vi "PH_Timing.set Default.vi"(0 "i ref in":refnum<vi>, 5 "error in (no error)":errorcluster) -> (14 "i ref out":refnum<vi>, 19 "error out":errorcluster)   [LabVIEW 2014, in "PH_Timing.lvlib"]
doc: "Within this VI the default settings are set to the GUI."
uses:
  PH_Timing.lvlib
  PH_Basics/PH_Common/PH_Common.lvlib
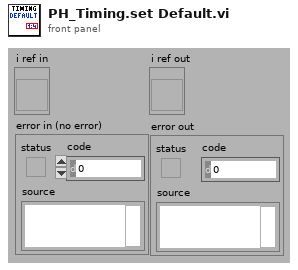
[diagram p1: front panel]
types:
  T1 = typedef "PH_Timing.lvlib/PH_Timing.i attribute.ctl" = cluster{"Sequencer":cluster{"linked?":bool, "Proc State":string, "Ref State":refnum<vi>}, "Gate Generator":cluster{"GD":cluster{"Device Status":T2, "linked?":bool}, "Settings":T3, "GUI Ref":refnum<vi>}, "Interlock Bypass":cluster{"Instancename":string, "Switch linked?":bool, "Device Status":T2, "Ref Status":refnum<vi>}, "Roughtuner":cluster{"Settings":T4, "GUI Ref":refnum<vi>, "GD":cluster{"Device Status":T2, "linked?":bool}}, "0,5Hz Gater":cluster{"Settings":T5, "GUI Ref":refnum<vi>, "GD":cluster{"Device Status":T2, "linked?":bool}}, "Slow Trigger":cluster{"Settings":T6, "GUI Ref":refnum<vi>, "Service ID Delay":i32, "Service ID Ext Trig":i32, "Wanted Settings":T6}, "Timing Mode":cluster{"Mode":T7, "GUI Ref":refnum<vi>, "Service ID T2":i32, "Service ID Mode":i32, "Wanted Mode":T7}, "ns Generator":cluster{"Settings":T8, "ns Generator Settings":refnum<vi>, "GD":cluster{"Device Status":T2, "linked?":bool}}, "Phase FEs":cluster{"Settings":T11, "GUI Ref":refnum<vi>, "Service ID Phase":i32, "Wanted Settings":T11}, "GD GUI Refs":refnum<vi>[], "Heads":T12[], "GUI Ref Delete":refnum<vi>}
  T2 = typedef "PH_StatusHandler.lvlib/PH_StatusHandler.Status.ctl" = i16
  T3 = typedef "PH_Timing.lvlib/PH_Timing.GateGen.ctl" = cluster{"Instance":string, "Channel Gate":i32, "Channel T2":i32, "Width Gate":dbl, "Width T2":dbl, "Delay Gate":dbl, "Delay T2":dbl, "Gate activ":bool, "T2 activ":bool, "System Mode":enum16{"Normal", "Single", "Burst", "Duty Cycle"}}
  T4 = typedef "PH_Timing.lvlib/PH_Timing.Roughtuner.ctl" = cluster{"Instance":string, "Phase PHELIX / UNILAC":cluster{"Channel":u16, "relative to":u16, "Delay [ms]":dbl}, "Pulse Length":cluster{"Channel":u16, "relative to":u16, "Delay [ms]":dbl}, "Trigger":cluster{"externally?":bool, "Rate [Hz]":dbl}}
  T5 = typedef "PH_Timing.lvlib/PH_Timing.0.5HzGater.ctl" = cluster{"Instance":string, "Channel ns FE Delay":i32, "Channel 0.5Hz":i32, "Width ns FE Delay":dbl, "Width 0.5Hz":dbl, "Delay ns FE Delay":dbl, "Delay 0.5Hz":dbl, "ns FE Delay active":bool, "0.5Hz activ":bool, "ns FE Delay inverted":bool, "0.5Hz inverted":bool}
  T6 = typedef "PH_Timing.lvlib/PH_Timing.Slow Trigger Settings.ctl" = cluster{"Delay":dbl, "externally triggered?":bool}
  T7 = typedef "PH_Timing.lvlib/PH_Timing.Timing Mode.ctl" = cluster{"T2":i16, "Modeselector":enum32{"10 Hz", "0.5 Hz", "Shot"}}
  T8 = typedef "PH_Timing.lvlib/PH_Timing.ns Generator.ctl" = cluster{"Instance":string, "Phase fs / ns FE":cluster{"Channel":T9, "Settings":T10}}
  T9 = typedef "Stanford Research DG645 - Driver.lvlib/Channel.ctl" = i32
  T10 = typedef "PH_SRDG645.lvlib/PH_SRDG645.Channel Settings.ctl" = cluster{"Delay [s]":dbl, "relative to":i32}
  T11 = typedef "PH_Timing.lvlib/PH_Timing.Phase FEs.ctl" = cluster{"Phase":dbl}
  T12 = typedef "PH_Timing.lvlib/PH_Timing.PU Data.ctl" = cluster{"linked?":bool, "Data":T13, "GD":cluster{"Device Status":T2, "linked?":bool}, "GUI Ref":refnum<vi>, "PU":T14}
  T13 = typedef "PH_Timing.lvlib/PH_Timing.PU Info.ctl" = cluster{"Act CH?":bool, "GD":string, "CH":i32, "Delay":dbl, "active":bool, "in Use?":bool}
  T14 = typedef "PH_PP_Common.lvlib/PH_PP_Common.PUs.ctl" = enum16{"no Info", "PA-19mm-1", "PA-19mm-2", "PA-45mm-PILC", "PA-45mm-MAIN", "MA-PU-1", "MA-PU-2", "MA-PU-3", "MA-PU-4", "MA-PU-5", "MA-PU-6", "MA-FR", "MA-PILC", "PA-45mm-DP"}
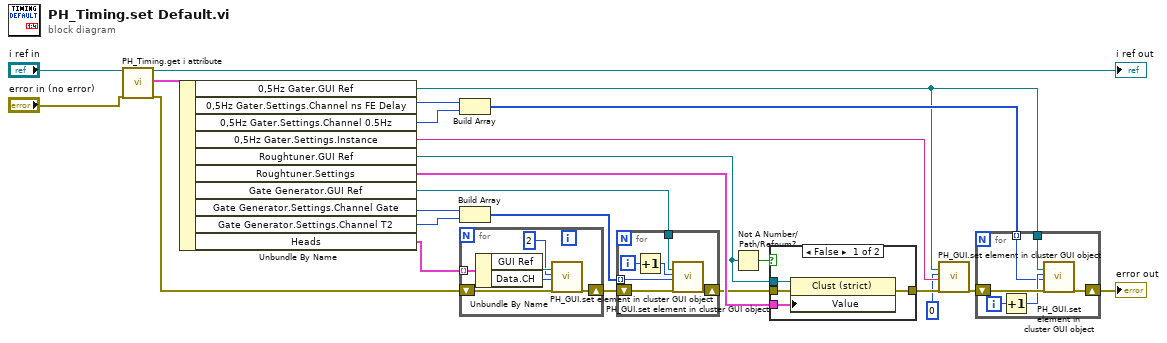
[diagram p0: block diagram]
diagram:
  n1 = call "PH_Timing.get i attribute.vi"("i ref in"="i ref in", "error in (no error)"="error in (no error)") -> ("i ref out"=→"i ref out":refnum<vi>, "i attribute"=w22:T1, "error out"=w21:errorcluster)  [unwired: 15 in]
  n2 = Unbundle By Name(w22) -> ("0,5Hz Gater.GUI Ref"=w5:refnum<vi>, "0,5Hz Gater.Settings.Channel ns FE Delay"=w9:i32, "0,5Hz Gater.Settings.Channel 0.5Hz"=w8:i32, "0,5Hz Gater.Settings.Instance"=w7:string, "Roughtuner.GUI Ref"=w14:refnum<vi>, "Roughtuner.Settings"=w15:T4, "Gate Generator.GUI Ref"=w19:refnum<vi>, "Gate Generator.Settings.Channel Gate"=w18:i32, "Gate Generator.Settings.Channel T2"=w2:i32, "Heads"=w1:T12[])
  n3 = Build Array(w9, w8) -> (w6:i32[])
  n4 = Build Array(w18, w2) -> (w17:i32[])
  n5 = for {
    tunnel: w1 -> [w30] mode=indexing
    shift-right: [w26] -> w20
    shift-left: w21 -> [w25]
    n6 = Unbundle By Name(w30) -> ("GUI Ref"=w29:refnum<vi>, "Data.CH"=w28:i32)
    n7 = call "PH_GUI.set element in cluster GUI object.vi"("Cluster Ref"=w29, "Cluster index"=2, "Value"=w28, "error in (no error)"=w25) -> ("error out"=w26:errorcluster)  [unwired: 15 in]
  }
  n8 = for {
    shift-right: [w36] -> w3
    shift-left: w20 -> [w35]
    tunnel: w19 -> [w32]
    tunnel: w17 -> [w31] mode=indexing
    i -> [w34]
    n9 = Increment(x=w34) -> (x+1=w33:i32)
    n10 = call "PH_GUI.set element in cluster GUI object.vi"("Cluster Ref"=w32, "Cluster index"=w33, "Value"=w31, "error in (no error)"=w35) -> ("error out"=w36:errorcluster)  [unwired: 15 in]
  }
  n11 = Not A Number/Path/Refnum?(number/path/refnum=w14) -> (NaN/Path/Refnum?=w13:bool)
  n12 = case shown="False" w13 {
    tunnel: w14 -> [w37 _]
    tunnel: w15 -> [w39 _]
    tunnel: w3 -> [w38 w41]
    tunnel: [w40 w41] -> w10
    frame False {
      n13 = property class="Clust (strict)"(reference=w37, error in=w38, "Value"=w39) -> (error out=w40:errorcluster)  [unwired: 1 out]
    }
    frame True {
    }
  }
  n14 = call "PH_GUI.set element in cluster GUI object.vi"("Cluster Ref"=w5, "Cluster index"=0, "Value"=w7, "error in (no error)"=w10) -> ("error out"=w12:errorcluster)  [unwired: 15 in]
  n15 = for {
    shift-right: [w46] -> w11
    shift-left: w12 -> [w47]
    tunnel: w6 -> [w43] mode=indexing
    tunnel: w5 -> [w42]
    i -> [w44]
    n16 = Increment(x=w44) -> (x+1=w45:i32)
    n17 = call "PH_GUI.set element in cluster GUI object.vi"("Cluster Ref"=w42, "Cluster index"=w45, "Value"=w43, "error in (no error)"=w47) -> ("error out"=w46:errorcluster)  [unwired: 15 in]
  }
  "error out" <- w11
